vi "Sample Push Publish Sample Push ON.vi"(8 "error in (no error)":errorcluster, 10 "Sample Push ON":bool) -> (0 "error out":errorcluster)   [LabVIEW 2015, in "cRIO-Carbondioxide.lvlib" / "cRIO-CO2.lvlib" / "cRIO-CO2.lvclass"]
uses:
  cRIO-CO2.lvclass
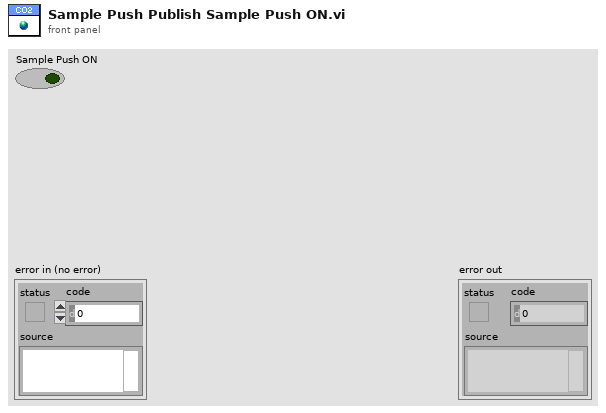
[diagram p1: front panel]
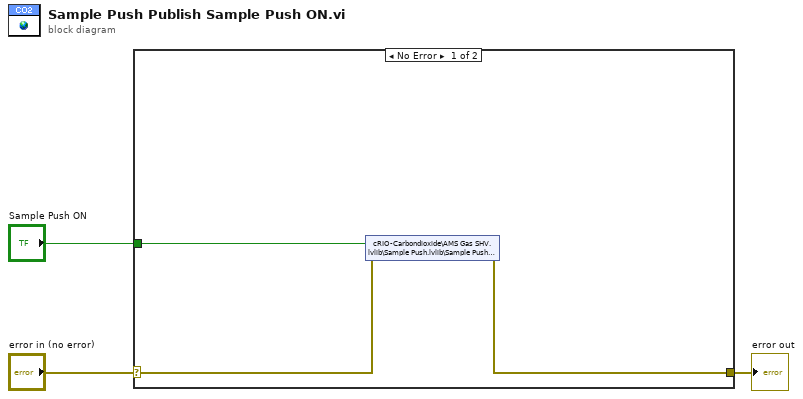
[diagram p0: block diagram]
diagram:
  n1 = case shown="No Error" "error in (no error)" {
    selector: "error in (no error)" -> [w6 w7]
    tunnel: [w5 w7] -> w2
    tunnel: "Sample Push ON" -> [w4 _]
    frame No Error {
      n2 = shared-variable "cRIO-Carbondioxide\\AMS Gas SHV.lvlib\\Sample Push.lvlib\\Sample Push ON"(w4, error in=w6) -> (error out=w5:errorcluster)
    }
    frame Error {
    }
  }
  "error out" <- w2
